vi "Estilos Labview.vi"() -> ()   [LabVIEW 2020]
panel:
  in  "String 6":string
  out "Boolean 6":bool
  in  "Numeric 6":dbl
  in  "Array 4":void[](array[numeric])
  in  "String 5":string
  out "Boolean 4":bool
  in  "Numeric 5":dbl
  out "Boolean 5":bool
  in  "String 4":string
  in  "Numeric 4":dbl
  in  "Array 3":void[](array[numeric])
  in  "String 3":string
  out "Boolean 3":bool
  in  "Numeric 3":dbl
  in  "Array 2":void[](array[numeric])
  in  "String 2":string
  out "Boolean 2":bool
  in  "Numeric 2":dbl
  in  "Array":void[](array[numeric])
  in  "String":string
  out "Boolean":bool
  in  "Numeric":dbl
  # "Tipo Modern"
  # "Tipo Classic"
  # "Tipo NXG Style"
  # "Tipo System"
  # "Tipo Silver"
  # "Tipo Express"
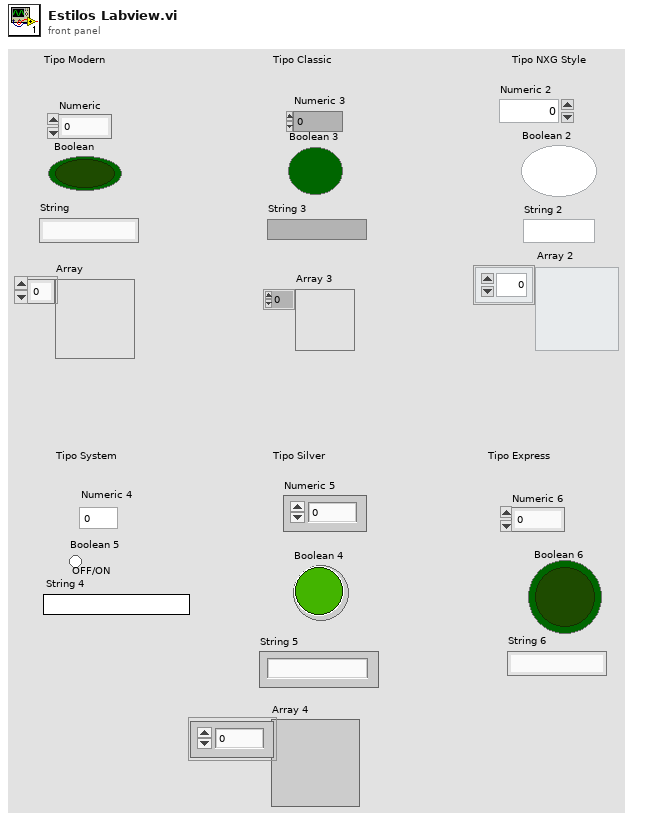
[diagram p1: front panel]
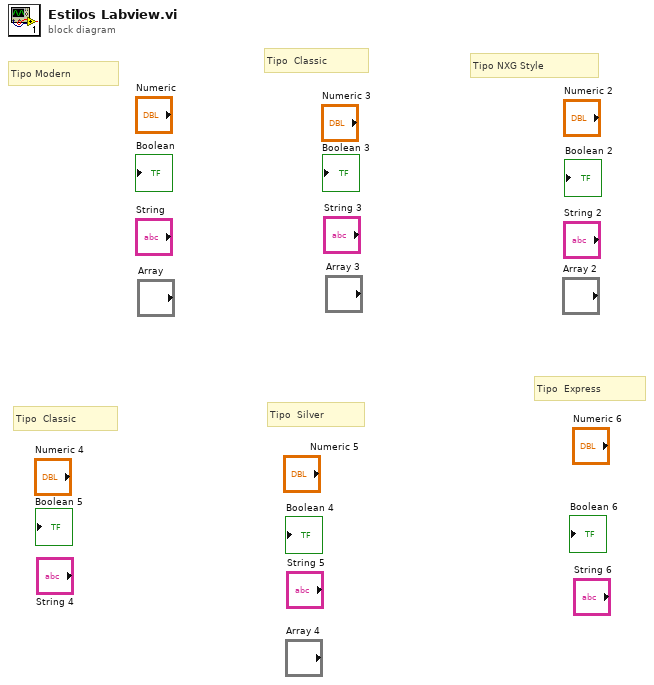
[diagram p0: block diagram]
diagram:
  # "Tipo  Express"
  # "Tipo  Silver"
  # "Tipo  Classic"
  # "Tipo  Classic"
  # "Tipo NXG Style"
  # "Tipo Modern"
